vi "PH_Cont-601k_PSU.PC Voltage.vi"(0 "VI in":refnum<vi>, 2 "Voltage [V]":u16, 5 "error in (no error)":errorcluster) -> (14 "VI out":refnum<vi>, 17 "\"Voltage\" changed":bool, 19 "error out":errorcluster)   [LabVIEW 2014, in "PH_Cont-601k_PSU.lvlib"]
uses:
  PH_Cont-601k_PSU.lvlib
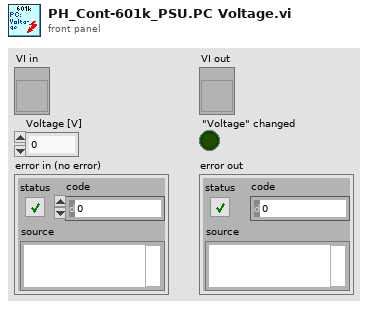
[diagram p1: front panel]
types:
  T1 = typedef "PH_Cont-601k_PSU.lvlib/PH_Cont-601k_PSU.i attribute.ctl" = cluster{"GUI Refs":T2, "Interlock":bool, "Service ID applied Voltage":i32, "Device Settings":cluster{"Configuration":T3, "Flash Interval [s]":dbl, "Mode":T4, "Voltage [V]":u16, "Charge":bool, "VISA resource name":refnum<visa-resource-name>}, "Readyness":T5, "Information":cluster{"VISA resource name":refnum<visa-resource-name>, "Tagname Power On":string, "Interlock":cluster{"Instance":string, "Tagname":string}, "Limits [V]":cluster{"Lower":dbl, "Upper":dbl}, "Tagname PSU On":string}, "R2S":bool, "Charge is allowed":bool}
  T2 = typedef "PH_Cont-601k_PSU.lvlib/PH_Cont-601k_PSU.GUI Refs.ctl" = cluster{"Power On":refnum<vi>, "Hard- and Software":refnum<vi>, "Device Status":refnum<vi>, "Device Error":refnum<vi>, "Configuration":refnum<vi>, "Flash Interval [s]":refnum<vi>, "Interlock":refnum<vi>, "Interlock Indicator":refnum<vi>, "Voltage [V]":refnum<vi>, "Readyness":refnum<vi>, "Mode":refnum<vi>, "Reset Error":refnum<vi>, "Expert working":refnum<vi>, "Charge":refnum<vi>, "PSU On":refnum<vi>}
  T3 = typedef "PH_Cont-601k_PSU.lvlib/PH_Cont-601k_PSU.Configuration.ctl" = u16
  T4 = typedef "PH_Cont-601k_PSU.lvlib/PH_Cont-601k_PSU.Mode.ctl" = enum32{"STOP", "STANDBY", "READY", "EMISSION", "ERROR"}
  T5 = typedef "PH_Cont-601k_PSU.lvlib/PH_Cont-601k_PSU.Readyness.ctl" = cluster{"Program":T6, "Device":T7}
  T6 = typedef "PH_Cont-601k_PSU.lvlib/PH_Cont-601k_PSU.Readyness Program.ctl" = enum32{"OFF", "POWER", "INTERLOCK"}
  T7 = typedef "PH_Cont-601k_PSU.lvlib/PH_Cont-601k_PSU.Readyness Device.ctl" = enum32{"OFF", "CONNECTING", "CONNECTED", "OPERATING", "EOC", "ERROR"}
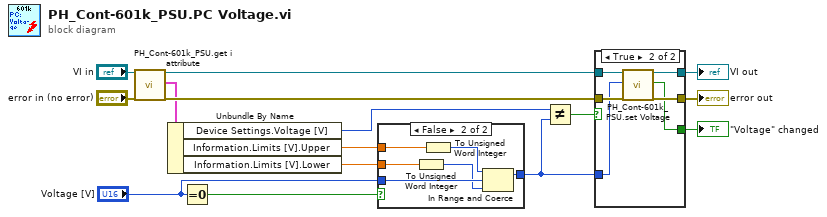
[diagram p0: block diagram]
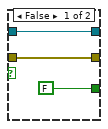
[diagram p2: hidden frame]
diagram:
  n1 = call "PH_Cont-601k_PSU.get i attribute.vi"("i ref in"="VI in", "error in (no error)"="error in (no error)") -> ("i ref out"=w12:refnum<vi>, "i attribute"=w9:T1, "error out"=w13:errorcluster)  [unwired: 15 in]
  n2 = Unbundle By Name(w9) -> ("Device Settings.Voltage [V]"=w8:u16, "Information.Limits [V].Upper"=w4:dbl, "Information.Limits [V].Lower"=w3:dbl)
  n3 = Equal To 0?(x="Voltage [V]") -> (x = 0?=w11:bool)
  n4 = case shown="False" w11 {
    tunnel: "Voltage [V]" -> [w16 w22]
    tunnel: [w16 w21] -> w7
    tunnel: w4 -> [_ w20]
    tunnel: w3 -> [_ w19]
    frame True {
    }
    frame False {
      n5 = To Unsigned Word Integer(number=w19) -> (unsigned 16bit integer=w18:u16)
      n6 = To Unsigned Word Integer(number=w20) -> (unsigned 16bit integer=w17:u16)
      n7 = In Range and Coerce(upper limit=w17, x=w22, lower limit=w18) -> (coerced(x)=w21:u16)  [unwired: 1 out]
    }
  }
  n8 = Not Equal?(x=w8, y=w7) -> (x != y?=w6:bool)
  n9 = case shown="True" w6 {
    tunnel: [w25 w31] -> w15
    tunnel: [w24 w30] -> w14
    tunnel: w13 -> [w24 w29]
    tunnel: w12 -> [w25 w28]
    tunnel: w7 -> [_ w27]
    tunnel: [FALSE w26] -> w5
    frame False {
    }
    frame True {
      n10 = call "PH_Cont-601k_PSU.set Voltage.vi"("VI in"=w28, "Voltage [V]"=w27, "error in (no error)"=w29) -> ("VI out"=w31:refnum<vi>, "Voltage changed"=w26:bool, "error out"=w30:errorcluster)  [unwired: 14 in]
    }
  }
  "VI out" <- w15
  "error out" <- w14
  "\"Voltage\" changed" <- w5
